vi "Servo Turn off unnecessary drive.vi"(8 "error in (no error)":errorcluster, 9 "Status now":T1, 10 "Status before":T1, 11 "Connection":variant) -> (0 "error out":errorcluster, 2 "Status out":T1)   [LabVIEW 2022 SP3, in "Servo drive module.lvlib"]
doc: "Turns off drives, that are at target. (debounced)"
uses:
  Servo drive module.lvlib
  ctl/Servo variables.ctl
  <vilib>/addons/eal4LabVIEW/eal4LabVIEW.lvlib
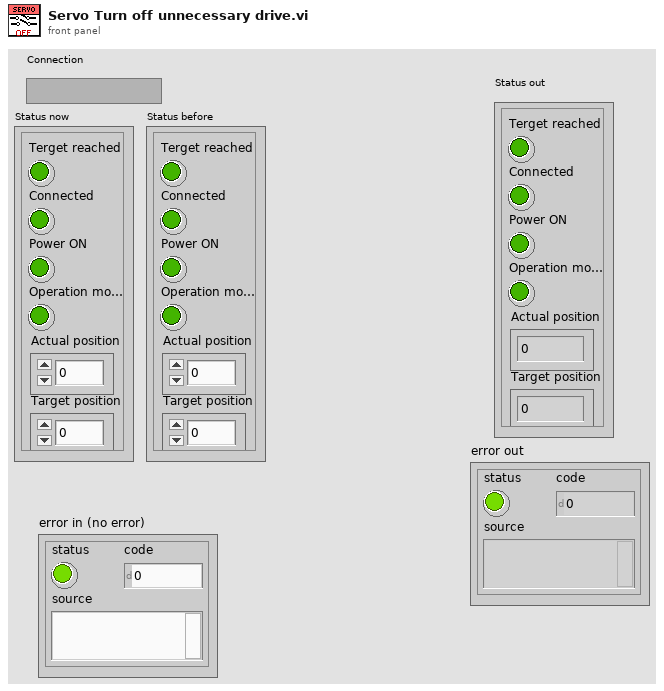
[diagram p1: front panel]
types:
  T1 = typedef "Servo drive module.lvlib/Servo variables.ctl" = cluster{"Terget reached":bool, "Connected":bool, "Power ON":bool, "Operation mode":bool, "Actual position":dbl, "Target position":dbl}
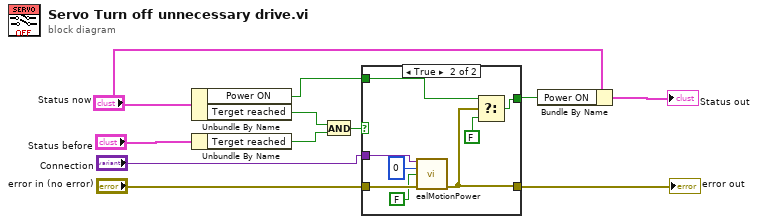
[diagram p0: block diagram]
diagram:
  n1 = Unbundle By Name("Status now") -> ("Power ON"=w6:bool, "Terget reached"=w1:bool)
  n2 = Unbundle By Name("Status before") -> ("Terget reached"=w8:bool)
  n3 = And(x=w1, y=w8) -> (x .and. y?=w3:bool)
  n4 = case shown="True" w3 {
    tunnel: "error in (no error)" -> [w13 w21]
    tunnel: [w13 w17] -> w10
    tunnel: "Connection" -> [_ w18]
    tunnel: w6 -> [w12 w14]
    tunnel: [w12 w15] -> w5
    frame False {
    }
    frame True {
      n5 = call <vilib>:"ealMotionPower.vi"("connection in"=w18, "slave index"=0, "value"=FALSE, "error in (no error)"=w21) -> ("error out"=w17:errorcluster)  [unwired: 10 in, 1 out]
      n6 = Select(t=w14, s=w17, f=FALSE ("Boolean")) -> (s? t:f=w15:bool)
    }
  }
  "error out" <- w10
  n7 = Bundle By Name(cluster="Status now", "Power ON"=w5) -> (→"Status out":T1)
